vi "RX_多通道FM.vi"() -> ()   [LabVIEW 2019]
uses:
  <instrlib>/niUSRP/niUSRP Fetch Rx Data (CDB WDT).vi
  <vilib>/express/express analysis/Spectral/Block/exnSpectralBlock spectral measurements RMS poly.vi
  <vilib>/express/express analysis/Spectral/Block/exnSpectralBlock spectral measurements RMS WFM.vi
  <vilib>/addons/Modulation/Analog/MT Passband PLL.vi
  <vilib>/Analysis/2dsp.llb/Rational Resample (single channel, DBL).vi
  <vilib>/sound2/lvsound2.llb/Sound Output Write (DBL Single).vi
  <vilib>/express/express analysis/Spectral/XNode/ExpressSpectralMeasurementsBlockNode.xnode
  <vilib>/Analysis/NI_AALPro.lvlib
  <vilib>/addons/Modulation/niAMT.lvlib
panel:
  out "estimated carrier frequency (Hz) 2":dbl caption="estimated carrier frequency (Hz)"
  out "estimated carrier frequency (Hz)":dbl
  out "specture 2":cluster{"f0":dbl, "df":dbl, "magnitude":dbl[]}(graph)
  in  "Lower Cut-Off":dbl=100000.0
  in  "resample rate":dbl=1000000.0 format="%#_13g"
  out "error out 2":errorcluster
  in  "Sound format":T1={"sample rate(S/s)"=44100.0, "number of samples"=1.0, "bits per sample"=16.0}
  out "error out":errorcluster
  in  "stop":bool
  out "XY Graph":cluster{dbl[], dbl[]}(graph)
  out "specture":cluster{"f0":dbl, "df":dbl, "magnitude":dbl[]}(graph)
  in  "device names":refnum<k15>="192.168.10.2"
  in  "active antenna":string="RX2"
  out "c gain":dbl
  out "coerced carrier frequency":dbl=2400000000.0
  out "coerced IQ rate":dbl=200000.0
  in  "gain":dbl
  in  "Carrier frequency":dbl=2400000000.0
  in  "IQ rate":dbl=200000.0
  in  "number fo samples":i64=44100
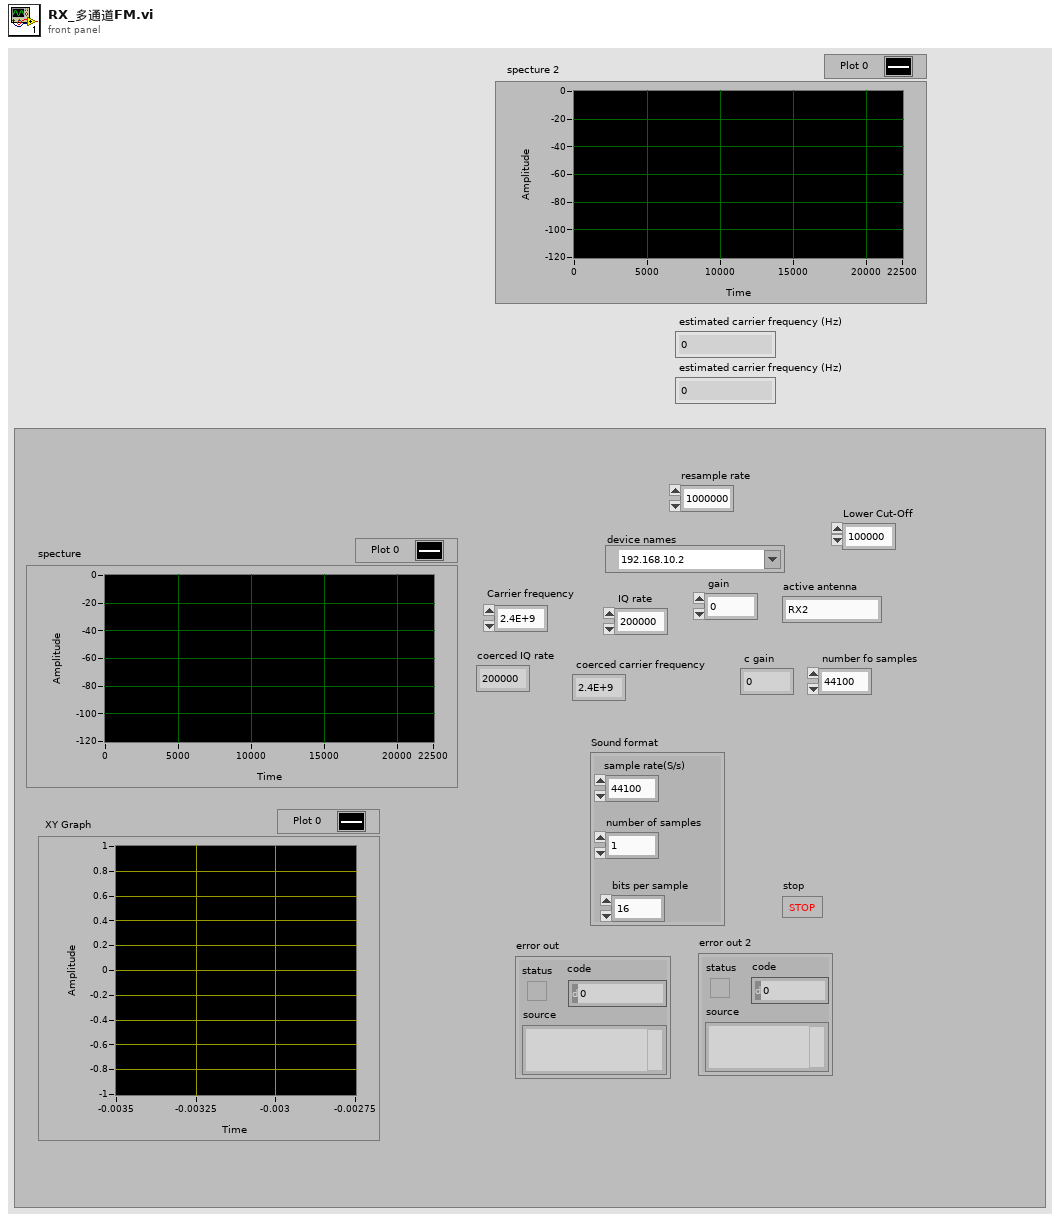
[diagram p1: front panel]
types:
  T1 = cluster{"sample rate(S/s)":dbl, "number of samples":dbl, "bits per sample":dbl}
  T2 = typedef "Sound Output Task ID.ctl" = u32
  T3 = cluster{"averaging mode":u16, "weighting mode":u16, "number of averages":u32}
  T4 = cluster{"dB On (F)":bool, "unwrap phase (F)":bool, "convert to degree (F)":bool}
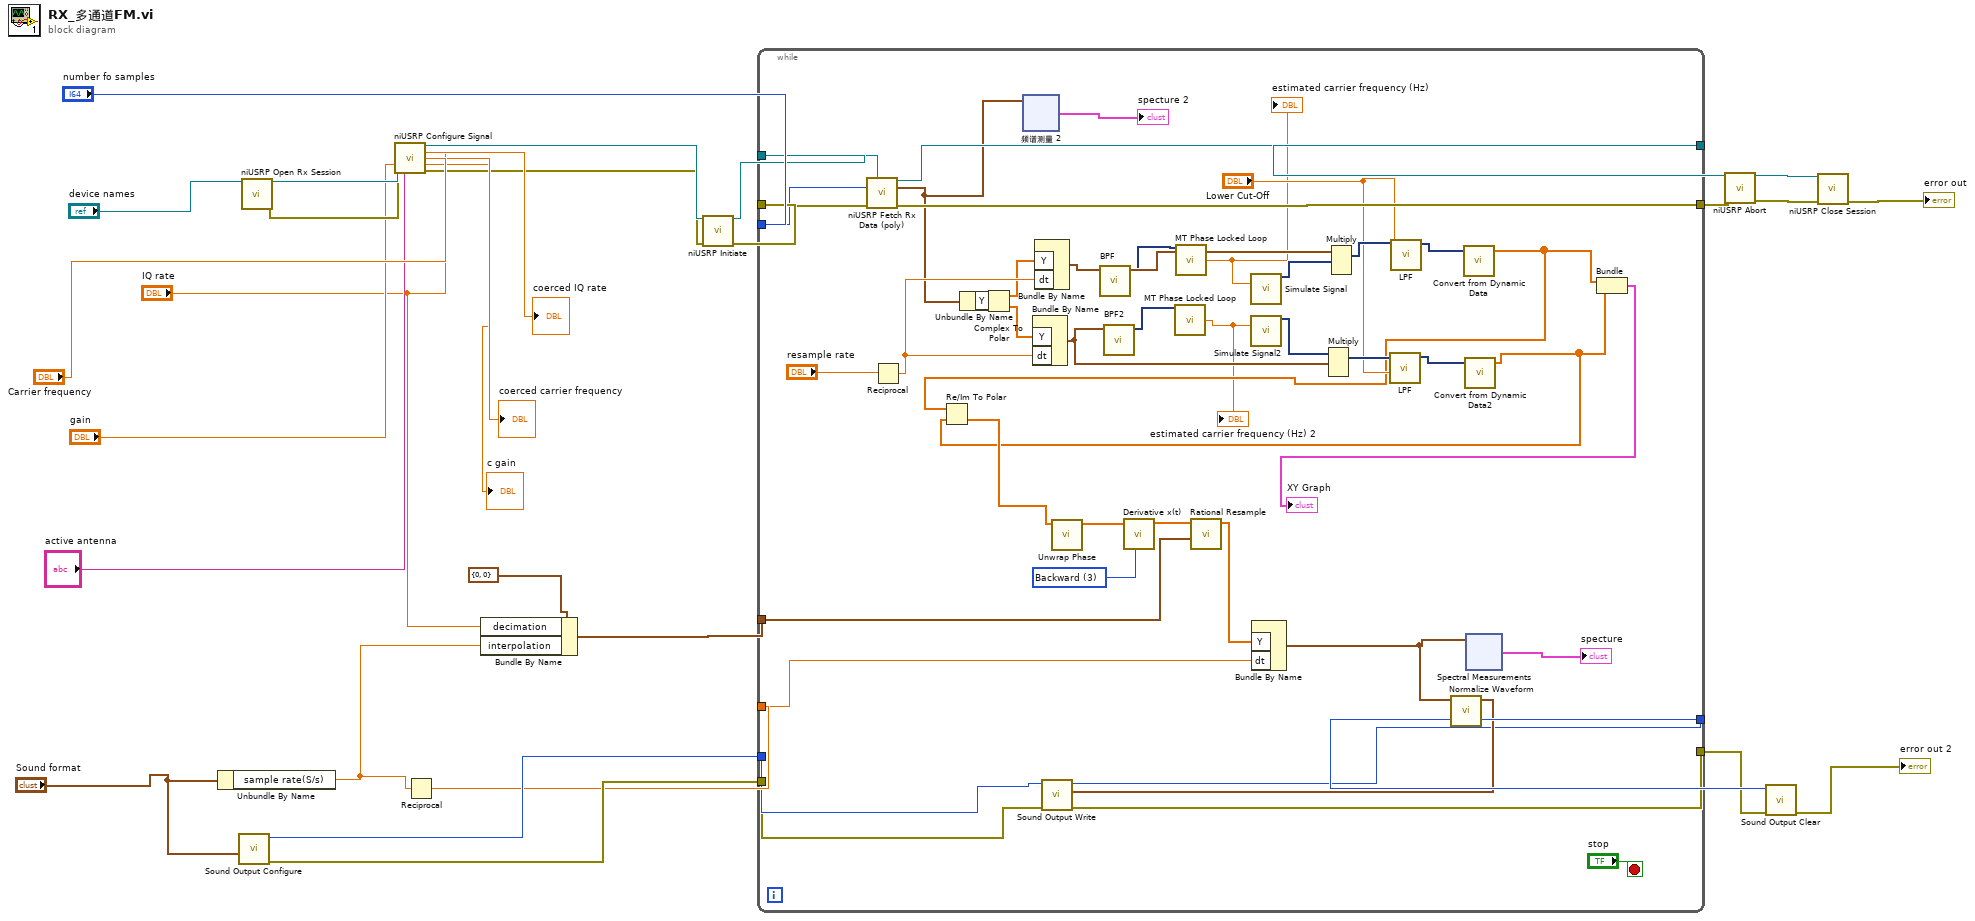
[diagram p0: block diagram]
diagram:
  n1 = Unbundle By Name("Sound format") -> ("sample rate(S/s)"=w6:dbl)
  n2 = call <vilib>:"Sound Output Configure.vi"("sound format"="Sound format") -> ("error out"=w11:errorcluster, "task ID"=w12:T2)  [unwired: 9 in]
  n3 = call <instrlib>:"niUSRP Open Rx Session.vi"("device names"="device names") -> ("session handle out"=w30:refnum<k15>, "error out"=w22:errorcluster)  [unwired: 13 in]
  n4 = call <instrlib>:"niUSRP Configure Signal.vi"("session handle"=w30, "IQ rate"="IQ rate", "carrier frequency"="Carrier frequency", "gain"="gain", "error in (no error)"=w22, "active antenna"="active antenna") -> ("session handle out"=w23:refnum<k15>, "coerced IQ rate"=→"coerced IQ rate":dbl, "coerced carrier frequency"=→"coerced carrier frequency":dbl, "coerced gain"=→"c gain":dbl, "error out"=w21:errorcluster)  [unwired: 5 in]
  n5 = Reciprocal(x=w6) -> (1/x=w5:dbl)
  n6 = Bundle By Name(cluster=cluster{"interpolation":i32, "decimation":i32} {"interpolation"=0, "decimation"=0} ("input cluster"), "decimation"="IQ rate", "interpolation"=w6) -> (w13:cluster{"interpolation":i32, "decimation":i32})
  n7 = call <instrlib>:"niUSRP Initiate.vi"("session handle"=w23, "error in (no error)"=w21) -> ("session handle out"=w19:refnum<k15>, "error out"=w4:errorcluster)  [unwired: 12 in]
  n8 = while {
    tunnel: "number fo samples" -> [w73]
    tunnel: [w53] -> w18
    tunnel: w19 -> [w72]
    tunnel: w13 -> [w68]
    tunnel: w12 -> [w62]
    tunnel: w11 -> [w61]
    tunnel: w5 -> [w65]
    tunnel: [w60] -> w8
    tunnel: [w59] -> w9
    tunnel: w4 -> [w58]
    tunnel: [w57] -> w3
    stop <- "stop" stop-if-true
    w67 = u16 3 items=["2nd Order Central", "4th Order Central", "Forward", "Backward"] ("method")
    n9 = call-poly <instrlib>:"niUSRP Fetch Rx Data (poly).vi"("session handle"=w72, "number of samples"=w73, "error in (no error)"=w58) -> ("session handle out"=w53:refnum<k15>, "data"=w37:waveform(cdb), "error out"=w57:errorcluster)  [unwired: 9 in, 1 out]
    n10 = Reciprocal(x="resample rate") -> (1/x=w51:dbl)
    n11 = Unbundle By Name(w37) -> ("Y"=w52:cdb[])
    n12 = Complex To Polar(r * e^(i*theta)=w52) -> (r=w50:dbl[], theta=w49:dbl[])
    n13 = xnode "频谱测量 2"("信号"=w37) -> ("FFT - (RMS)"=→"specture 2":cluster{"f0":dbl, "df":dbl, "magnitude":dbl[]})  [unwired: 1 in, 2 out]
    n14 = Bundle By Name("Y"=w49, "dt"=w51) -> (w35:waveform(dbl))  [unwired: 1 in]
    n15 = Bundle By Name("Y"=w50, "dt"=w51) -> (w36:waveform(dbl))  [unwired: 1 in]
    n16 = call "BPF"("Signal"=w36) -> ("Filtered Signal"=w34:dynamicdata)  [unwired: 9 in, 1 out]
    n17 = call "BPF2"("Signal"=w35) -> ("Filtered Signal"=w32:dynamicdata)  [unwired: 9 in, 1 out]
    n18 = call-poly <vilib>:"MT Phase Locked Loop.vi"("passband waveform"=w32) -> ("estimated carrier frequency (Hz)"=w31:dbl)  [unwired: 10 in, 4 out]
    "estimated carrier frequency (Hz) 2" <- w31
    n19 = call-poly <vilib>:"MT Phase Locked Loop.vi"("passband waveform"=w34) -> ("estimated carrier frequency (Hz)"=w33:dbl)  [unwired: 10 in, 4 out]
    "estimated carrier frequency (Hz)" <- w33
    n20 = call "Simulate Signal"("Frequency"=w33) -> ("正弦"=w48:dynamicdata)  [unwired: 13 in, 1 out]
    n21 = call "Simulate Signal2"("Frequency"=w31) -> ("Sine"=w47:dynamicdata)  [unwired: 13 in, 1 out]
    n22 = Multiply(1:w35, 2:w47) -> (0:w45:dynamicdata)  [unwired: 1 in, 1 out]
    n23 = Multiply(1:w48, 2:w36) -> (0:w46:dynamicdata)  [unwired: 1 in, 1 out]
    n24 = call "LPF"("Lower Cut-Off"="Lower Cut-Off", "Signal"=w45) -> ("Filtered Signal"=w42:dynamicdata)  [unwired: 8 in, 1 out]
    n25 = call "LPF"("Lower Cut-Off"="Lower Cut-Off", "Signal"=w46) -> ("Filtered Signal"=w43:dynamicdata)  [unwired: 8 in, 1 out]
    n26 = call "Convert from Dynamic Data"("Dynamic Data Type"=w43) -> ("Array"=w40:dbl[])  [unwired: 3 in]
    n27 = call "Convert from Dynamic Data2"("Dynamic Data Type"=w42) -> ("Array"=w39:dbl[])  [unwired: 3 in]
    n28 = Re/Im To Polar(2:w39, 3:w40) -> (0:w41:dbl[])  [unwired: 1 out]
    n29 = call <vilib>:"Unwrap Phase.vi"("Phase"=w41) -> ("Unwrapped Phase"=w70:dbl[])  [unwired: 9 in, 1 out]
    n30 = call <vilib>:"Derivative x(t).vi"("method"=w67, "X"=w70) -> ("dX/dt"=w69:dbl[])  [unwired: 8 in, 1 out]
    n31 = call-poly <vilib>:"Rational Resample.vi"("resample factor"=w68, "X"=w69) -> ("Y"=w66:dbl[])  [unwired: 7 in, 2 out]
    n32 = Bundle By Name("Y"=w66, "dt"=w65) -> (w64:waveform(dbl))  [unwired: 1 in]
    n33 = call <vilib>:"Normalize Waveform.vi"("waveform in"=w64) -> ("normalized waveform"=w63:waveform(dbl))  [unwired: 7 in, 3 out]
    n34 = call-poly <vilib>:"Sound Output Write.vi"("error in (no error)"=w61, "data"=w63, "task ID"=w62) -> ("error out"=w60:errorcluster, "task ID out"=w59:T2)  [unwired: 7 in]
    n35 = xnode "Spectral Measurements"("信号"=w64) -> ("FFT - (RMS)"=→"specture":cluster{"f0":dbl, "df":dbl, "magnitude":dbl[]})  [unwired: 1 in, 2 out]
    n36 = Bundle("Array"=w40, "Array"=w39) -> (→"XY Graph":cluster{"Array":dbl[], "Array":dbl[]})  [unwired: 1 in]
  }
  n37 = call <instrlib>:"niUSRP Abort.vi"("session handle"=w18, "error in (no error)"=w3) -> ("session handle out"=w17:refnum<k15>, "error out"=w16:errorcluster)  [unwired: 12 in]
  n38 = call <vilib>:"Sound Output Clear.vi"("error in (no error)"=w8, "task ID"=w9) -> ("error out"=→"error out 2":errorcluster)  [unwired: 9 in]
  n39 = call <instrlib>:"niUSRP Close Session.vi"("session handle"=w17, "error in (no error)"=w16) -> ("error out"=→"error out":errorcluster)  [unwired: 13 in]
